vi "AlliGator NLSF & Phasor Multi-ROI Analysis Dialog.vi"(0 "Dialog Type":T22, 11 "error in (no error)":errorcluster) -> (1 "Dataset Loading & Pre-processing Options":T3={"Data Information"={"Gates to Skip"={"Start"=0, "End"=0}, "# Gates"=1, "Gate Step"=1, "Gate Duration"=3e-10, "Gate Separation"=4e-11, "Pile-up Correction"=FALSE, "Pixel Well Capacity"=1, "Define Gates to"=enum."Skip", "Gates to Keep"={"First"=0, "Last"=0}, "Laser Period"=0.0, "SYNC Period"=0.0, "Channel Name"=0, "Channel Arithmetic"=enum."None", "Background File Subtraction"=FALSE, "Background Scaling Factor"=1.0, "Background File"=path "", "Background Pile-up Correction"=FALSE, "Background Pixel Well Capacity"=1, "Dataset Scaling Factor"=1.0}, "Source Image Settings"={"Low Count Pixels Rejection Options"={"Background Low Threshold Factor"=0.0, "Fixed Low Background Threshold"=20000.0, "Reject Low Count Pixels"=FALSE, "Low Percentile"=0.0}, "High Count Pixels Rejection Options"={"Background High Threshold Factor"=0.0, "Fixed High Background Threshold"=1.0, "Reject High Count Pixels"=FALSE, "High Percentile"=100.0}, "Peak Threshold"=500.0, "Intensity Threshold"=500.0, "Image Smoothing Options"={"Use Image Smoothing"=FALSE, "Kernel Type"=enum."Bilinear", "Bin"=1, "Algorithm"=enum."Rapid"}, "Image Binning Options"={"Use Image Binning"=FALSE, "X Bin"=1, "Y Bin"=1}}, "Decay Preprocessing Options & Parameters"={"Background Subtraction Parameters"={"Background Definition Range"={"Min Gate"=0.0, "Max Gate"=0.0}, "Baseline Subtraction Method"=enum."Mean", "Background Subtraction?"=FALSE, "Background File"=path "", "Background Constant"=0.0, "Background Scaling Factor"=1.0, "Background Pile-up Correction"=FALSE, "Background Pixel Well Capacity"=1}, "Decay Preprocessing Parameters"={"Background Subtraction"=FALSE, "Straighten Decay"=FALSE, "Reverse Gates"=FALSE, "1-Normalized Decay"=FALSE, "Smoothen Decay"=FALSE, "Smoothing Parameter"=0.0, "Shift Decay"=FALSE, "Decay Shift Parameters"={"Type"=enum."Default", "Shift"=0.0, "Threshold"=0.0, "Rotate"=FALSE}, "Extrapolate Decay"=FALSE, "Additional Points"=0, "Head Fraction"=0.0, "Pixel-Normalize Decay"=FALSE, "Use Periodicity"=FALSE, "Use Cursors"=FALSE, "Tail Fraction"=0.0, "Use Decay Pre-Processing"=TRUE, "Fold Decay"=FALSE, "# Folds"=1, "[0-1]-Normalized Decay"=FALSE}, "Preprocessing Steps Order"=[]}, "Clear Phasor Graph"=FALSE} {"Decay Preprocessing Options & Parameters"."Decay Preprocessing Parameters"."# Folds" min=1; "Decay Preprocessing Options & Parameters"."Background Subtraction Parameters"."Background Pixel Well Capacity" min=1 step=1; "Source Image Settings"."Image Binning Options"."Y Bin" min=1; "Source Image Settings"."Image Binning Options"."X Bin" min=1; "Source Image Settings"."Image Smoothing Options"."Bin" min=1; "Source Image Settings"."High Count Pixels Rejection Options"."High Percentile" min=0.0 max=100.0; "Source Image Settings"."Low Count Pixels Rejection Options"."Low Percentile" min=0.0 max=100.0; "Data Information"."Background Pixel Well Capacity" min=1 step=1; "Data Information"."Channel Name" items=["Bottom INT Gate", "Bottom G2 Gate"]; "Data Information"."SYNC Period" min=0.0 format="%#.3g"; "Data Information"."Laser Period" min=0.0 format="%#.3g"; "Data Information"."Pixel Well Capacity" min=1 step=1; "Data Information"."# Gates" min=1 step=1; "Data Information"."Gate Step" min=1 step=1; "Data Information"."Gate Duration" min=0.0 format="%#.3g"; "Data Information"."Gate Separation" min=0.0 format="%#.3g"}, 2 "IRF Loading & Pre-processing Options":T3={"Data Information"={"Gates to Skip"={"Start"=0, "End"=0}, "# Gates"=1, "Gate Step"=1, "Gate Duration"=3e-10, "Gate Separation"=4e-11, "Pile-up Correction"=FALSE, "Pixel Well Capacity"=1, "Define Gates to"=enum."Skip", "Gates to Keep"={"First"=0, "Last"=0}, "Laser Period"=0.0, "SYNC Period"=0.0, "Channel Name"=0, "Channel Arithmetic"=enum."None", "Background File Subtraction"=FALSE, "Background Scaling Factor"=1.0, "Background File"=path "", "Background Pile-up Correction"=FALSE, "Background Pixel Well Capacity"=1, "Dataset Scaling Factor"=1.0}, "Source Image Settings"={"Low Count Pixels Rejection Options"={"Background Low Threshold Factor"=0.0, "Fixed Low Background Threshold"=20000.0, "Reject Low Count Pixels"=FALSE, "Low Percentile"=0.0}, "High Count Pixels Rejection Options"={"Background High Threshold Factor"=0.0, "Fixed High Background Threshold"=1.0, "Reject High Count Pixels"=FALSE, "High Percentile"=100.0}, "Peak Threshold"=500.0, "Intensity Threshold"=500.0, "Image Smoothing Options"={"Use Image Smoothing"=FALSE, "Kernel Type"=enum."Bilinear", "Bin"=1, "Algorithm"=enum."Rapid"}, "Image Binning Options"={"Use Image Binning"=FALSE, "X Bin"=1, "Y Bin"=1}}, "Decay Preprocessing Options & Parameters"={"Background Subtraction Parameters"={"Background Definition Range"={"Min Gate"=0.0, "Max Gate"=0.0}, "Baseline Subtraction Method"=enum."Mean", "Background Subtraction?"=FALSE, "Background File"=path "", "Background Constant"=0.0, "Background Scaling Factor"=1.0, "Background Pile-up Correction"=FALSE, "Background Pixel Well Capacity"=1}, "Decay Preprocessing Parameters"={"Background Subtraction"=FALSE, "Straighten Decay"=FALSE, "Reverse Gates"=FALSE, "1-Normalized Decay"=FALSE, "Smoothen Decay"=FALSE, "Smoothing Parameter"=0.0, "Shift Decay"=FALSE, "Decay Shift Parameters"={"Type"=enum."Default", "Shift"=0.0, "Threshold"=0.0, "Rotate"=FALSE}, "Extrapolate Decay"=FALSE, "Additional Points"=0, "Head Fraction"=0.0, "Pixel-Normalize Decay"=FALSE, "Use Periodicity"=FALSE, "Use Cursors"=FALSE, "Tail Fraction"=0.0, "Use Decay Pre-Processing"=TRUE, "Fold Decay"=FALSE, "# Folds"=1, "[0-1]-Normalized Decay"=FALSE}, "Preprocessing Steps Order"=[]}, "Clear Phasor Graph"=FALSE} {"Decay Preprocessing Options & Parameters"."Decay Preprocessing Parameters"."# Folds" min=1; "Decay Preprocessing Options & Parameters"."Background Subtraction Parameters"."Background Pixel Well Capacity" min=1 step=1; "Source Image Settings"."Image Binning Options"."Y Bin" min=1; "Source Image Settings"."Image Binning Options"."X Bin" min=1; "Source Image Settings"."Image Smoothing Options"."Bin" min=1; "Source Image Settings"."High Count Pixels Rejection Options"."High Percentile" min=0.0 max=100.0; "Source Image Settings"."Low Count Pixels Rejection Options"."Low Percentile" min=0.0 max=100.0; "Data Information"."Background Pixel Well Capacity" min=1 step=1; "Data Information"."Channel Name" items=["Bottom INT Gate", "Bottom G2 Gate"]; "Data Information"."SYNC Period" min=0.0 format="%#.3g"; "Data Information"."Laser Period" min=0.0 format="%#.3g"; "Data Information"."Pixel Well Capacity" min=1 step=1; "Data Information"."# Gates" min=1 step=1; "Data Information"."Gate Step" min=1 step=1; "Data Information"."Gate Duration" min=0.0 format="%#.3g"; "Data Information"."Gate Separation" min=0.0 format="%#.3g"}, 3 "OK":bool, 4 "IRF File":path, 6 "Dataset File":path, 8 "ROI File":path, 10 "Decay Fit Parameters to Save":T23[](array[typedef]), 12 "Phasor Parameters Scatter Plots":T1[](array[typedef]), 13 "Bins Array":dbl[](array[numeric]), 14 "Results Folder":path, 15 "error out":errorcluster)   [LabVIEW 2021, in "AlliGator Scripts.lvlib"]
doc: "Dialog window to set up a multi-ROIs single-pixel NLSF analysis of a FLI dataset."
uses:
  AlliGator Scripts.lvlib
  Fits/IRF(X)PSED/Decay Fit Parameters & Derived Quantities List.ctl
  AlliGator Data Load & Process Options.ctl
  AlliGator Data Information.ctl
  AlliGator Gates to Skip.ctl
  AlliGator Define Gates to.ctl
  AlliGator Gates to Keep.ctl
  AlliGator Gate Arithmetic.ctl
  AlliGator Source Image Settings.ctl
  AlliGator Low Count Pixels Rejection Options.ctl
  AlliGator High Count Pixels Rejection Options.ctl
  AlliGator Image Smoothing Options.ctl
  Arrays/Kernel Type.ctl
  Arrays/Smoothing Algorithm.ctl
  AlliGator Image Binning Options.ctl
  AlliGator Decay Preprocessing Options.ctl
  AlliGator Background Subtraction Parameters.ctl
  AlliGator Baseline Subtraction Method.ctl
  AlliGator Decay Preprocessing Parameters.ctl
  Graphs/XY Graph/XY Graph Plot Shift Parameters.ctl
  Graphs/XY Graph/XY Graph Plot Shift Method.ctl
  AlliGator Multi-ROIs Dialog Type.ctl
  AlliGator Phasor Plot Scatter Plot Parameters.ctl
  AlliGator Phasor Graph Parameter List.ctl
  84fa21cc-6b70-40ff-a749-33f909e19637.vi
  Error/Error.lvlib
  Fits/Fits.lvlib
  AlliGator Decay Analysis.lvlib
  AlliGator Settings.lvlib
  Arrays/Arrays.lvlib
  AlliGator Source Image.lvlib
  AlliGator Decay Preprocessing.lvlib
  Graphs/XY Graph/XY Graph Add-Ons.lvlib
  AlliGator Phasor Graph.lvlib
panel:
  in  "Clear Phasor Graph":bool
  in  "Save Results":bool
  in  "Phasor Parameters Scatter Plots":T1[](array[typedef])
  in  "Tab Control":enum32{"IRF Options", "Dataset Options"}(tab)
  out "Dataset Settings Saved":bool
  in  "Set Dataset Parameters":bool
  in  "Save Script":bool
  in  "Load Script":bool
  out "IRF Settings Saved":bool
  out "Message":string
  in  "Set IRF Parameters":bool
  in  "Bins":dbl[](array[numeric])
  in  "Results Folder:":path caption="Dataset File"
  in  "Decay Fit Parameters to save:":T23[](array[typedef])
  in  "ROI File:":path caption="Dataset File"
  in  "Dataset File:":path caption="Dataset File"
  in  "IRF File:":path caption="IRF File"
  in  "Cancel":bool
  in  "Run Script":bool
  in  "Use IRF Dataset":bool
  # "vs"
  # "vs"
  # "Gates Characteristics"
  # "Background File Subtraction"
  # "Gates Characteristics"
  # "Background File Subtraction"
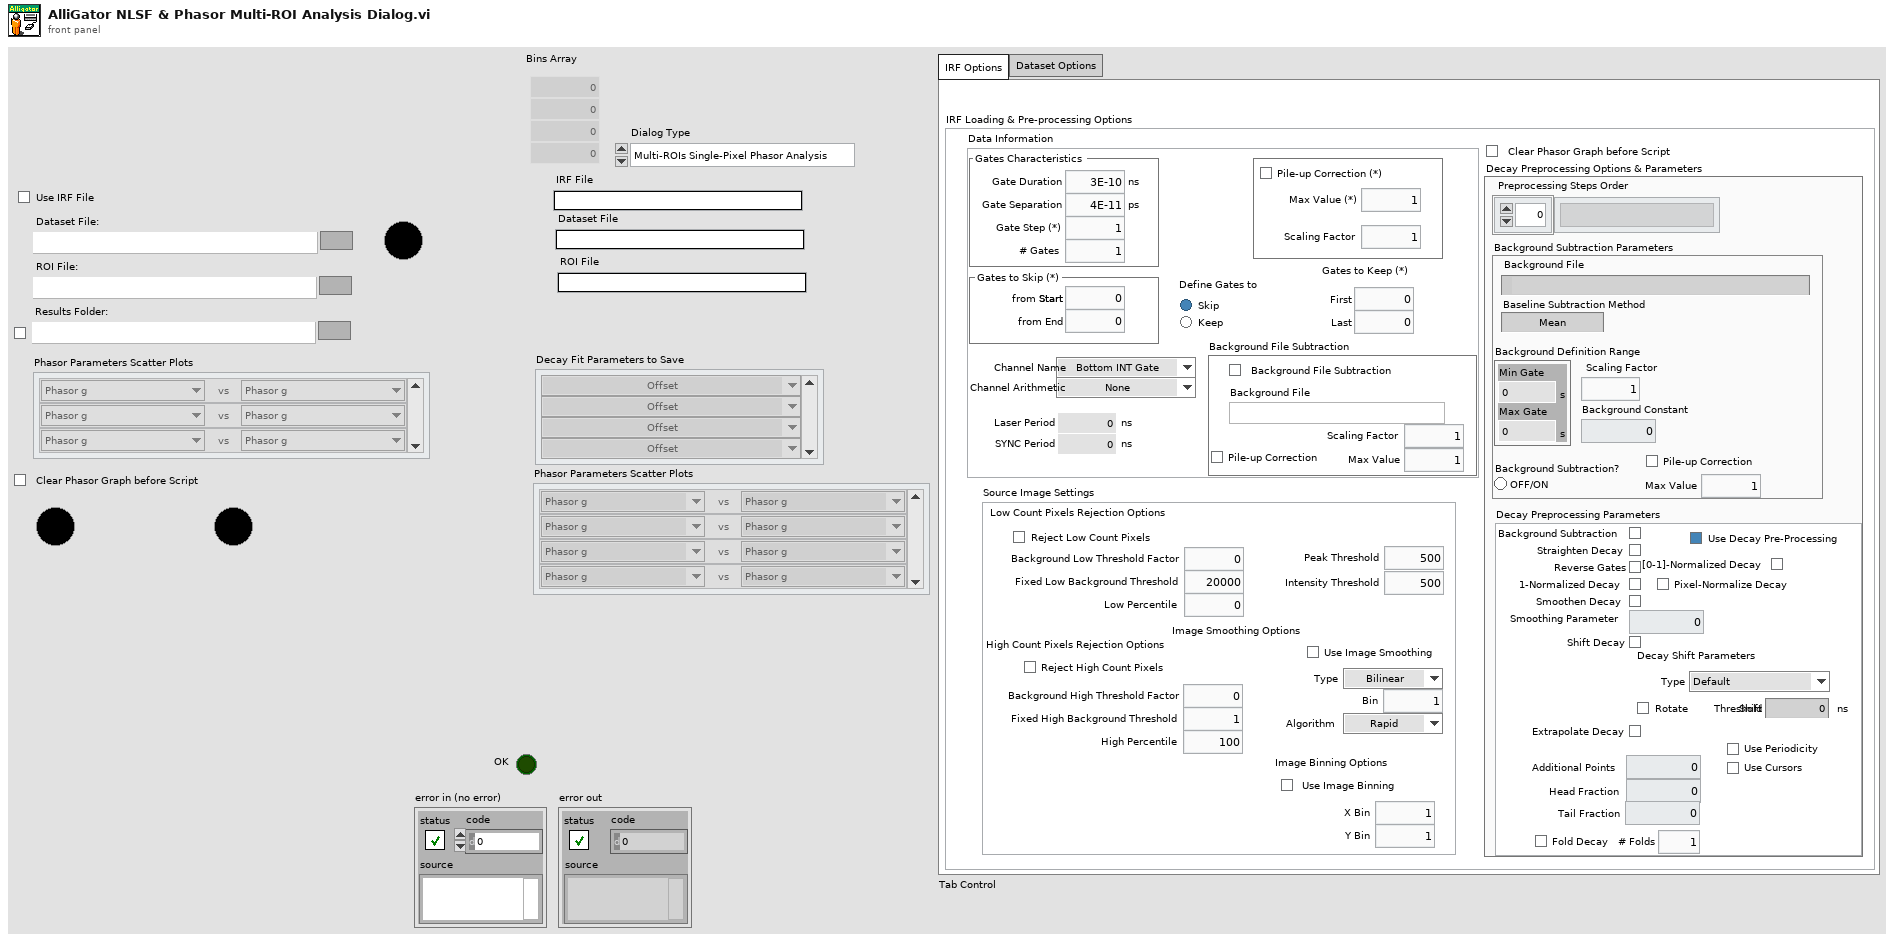
[diagram p1: front panel]
types:
  T1 = typedef "AlliGator Phasor Graph.lvlib/AlliGator Phasor Plot Scatter Plot Parameters.ctl" = cluster{"Parameter 2":T2, "Parameter 1":T2}
  T2 = typedef "AlliGator Phasor Graph.lvlib/AlliGator Phasor Graph Parameter List.ctl" = enum16{"Time Stamp", "Index", "Phasor Parameters", "Phasor g", "Phasor s", "Phasor phi", "Phasor m", "Modulus Lifetime", "Phase Lifetime", "ROI Parameters", "ROI Center x", "ROI Center y", "ROI # pixels ", "Decay Parameters", "Intensity", "Background/Gate", "Intensity - Background", "Fitted Lifetime", "Fitted Intensity", "Phasor Ratio Parameters", "Amplitude Phasor Ratio", "Intensity Phasor Ratio", "Amplitude-Averaged Lifetime", "Intensity-Averaged Lifetime", "-", "Phasor Parameters SDV", "Phasor g SDV", "Phasor s SDV", "Phasor phi SDV", "Phasor m SDV", "Phase Lifetime SDV", "Modulus Lifetime SDV", "Phasor Ratio Parameters SDV", "Amplitude Phasor Ratio SDV", "Intensity Phasor Ratio SDV", "Amplitude-Averaged Lifetime SDV", "Intensity-Averaged Lifetime SDV"}
  T3 = typedef "AlliGator Scripts.lvlib/AlliGator Data Load & Process Options.ctl" = cluster{"Data Information":T4, "Source Image Settings":T9, "Decay Preprocessing Options & Parameters":T16, "Clear Phasor Graph":bool}
  T4 = typedef "AlliGator Scripts.lvlib/AlliGator Data Information.ctl" = cluster{"Gates to Skip":T5, "# Gates":u32, "Gate Step":u32, "Gate Duration":dbl[unit], "Gate Separation":dbl[unit], "Pile-up Correction":bool, "Pixel Well Capacity":u32, "Define Gates to":T6, "Gates to Keep":T7, "Laser Period":dbl[unit], "SYNC Period":dbl[unit], "Channel Name":u16, "Channel Arithmetic":T8, "Background File Subtraction":bool, "Background Scaling Factor":dbl, "Background File":path, "Background Pile-up Correction":bool, "Background Pixel Well Capacity":u32, "Dataset Scaling Factor":dbl}
  T5 = typedef "AlliGator Decay Analysis.lvlib/AlliGator Gates to Skip.ctl" = cluster{"Start":u32, "End":u32}
  T6 = typedef "AlliGator Settings.lvlib/AlliGator Define Gates to.ctl" = enum32{"Skip", "Keep"}
  T7 = typedef "AlliGator Settings.lvlib/AlliGator Gates to Keep.ctl" = cluster{"First":u32, "Last":u32}
  T8 = typedef "AlliGator Settings.lvlib/AlliGator Gate Arithmetic.ctl" = enum16{"None", "INT-G2", "G2/INT*<INT>", "(1 - G2/INT)*<INT>"}
  T9 = typedef "AlliGator Scripts.lvlib/AlliGator Source Image Settings.ctl" = cluster{"Low Count Pixels Rejection Options":T10, "High Count Pixels Rejection Options":T11, "Peak Threshold":dbl, "Intensity Threshold":dbl, "Image Smoothing Options":T12, "Image Binning Options":T15}
  T10 = typedef "AlliGator Settings.lvlib/AlliGator Low Count Pixels Rejection Options.ctl" = cluster{"Background Low Threshold Factor":dbl, "Fixed Low Background Threshold":dbl, "Reject Low Count Pixels":bool, "Low Percentile":dbl}
  T11 = typedef "AlliGator Settings.lvlib/AlliGator High Count Pixels Rejection Options.ctl" = cluster{"Background High Threshold Factor":dbl, "Fixed High Background Threshold":dbl, "Reject High Count Pixels":bool, "High Percentile":dbl}
  T12 = typedef "AlliGator Settings.lvlib/AlliGator Image Smoothing Options.ctl" = cluster{"Use Image Smoothing":bool, "Kernel Type":T13, "Bin":i32, "Algorithm":T14}
  T13 = typedef "Arrays.lvlib/Kernel Type.ctl" = enum16{"Uniform", "Bilinear", "Gaussian"}
  T14 = typedef "Arrays.lvlib/Smoothing Algorithm.ctl" = enum16{"Rapid", "Thorough"}
  T15 = typedef "AlliGator Source Image.lvlib/AlliGator Image Binning Options.ctl" = cluster{"Use Image Binning":bool, "X Bin":i32, "Y Bin":i32}
  T16 = typedef "AlliGator Decay Analysis.lvlib/AlliGator Decay Preprocessing.lvlib/AlliGator Decay Preprocessing Options.ctl" = cluster{"Background Subtraction Parameters":T17, "Decay Preprocessing Parameters":T19, "Preprocessing Steps Order":string[]}
  T17 = typedef "AlliGator Decay Analysis.lvlib/AlliGator Decay Preprocessing.lvlib/AlliGator Background Subtraction Parameters.ctl" = cluster{"Background Definition Range":cluster{"Min Gate":dbl[unit], "Max Gate":dbl[unit]}, "Baseline Subtraction Method":T18, "Background Subtraction?":bool, "Background File":path, "Background Constant":dbl, "Background Scaling Factor":dbl, "Background Pile-up Correction":bool, "Background Pixel Well Capacity":u32}
  T18 = typedef "AlliGator Decay Analysis.lvlib/AlliGator Decay Preprocessing.lvlib/AlliGator Baseline Subtraction Method.ctl" = enum16{"Mean", "Min", "Square Gated Single-Exponential", "File", "Constant"}
  T19 = typedef "AlliGator Decay Analysis.lvlib/AlliGator Decay Preprocessing.lvlib/AlliGator Decay Preprocessing Parameters.ctl" = cluster{"Background Subtraction":bool, "Straighten Decay":bool, "Reverse Gates":bool, "1-Normalized Decay":bool, "Smoothen Decay":bool, "Smoothing Parameter":dbl, "Shift Decay":bool, "Decay Shift Parameters":T20, "Extrapolate Decay":bool, "Additional Points":u32, "Head Fraction":dbl, "Pixel-Normalize Decay":bool, "Use Periodicity":bool, "Use Cursors":bool, "Tail Fraction":dbl, "Use Decay Pre-Processing":bool, "Fold Decay":bool, "# Folds":u32, "[0-1]-Normalized Decay":bool}
  T20 = typedef "XY Graph Add-Ons.lvlib/XY Graph Plot Shift Parameters.ctl" = cluster{"Type":T21, "Shift":dbl[unit], "Threshold":dbl, "Rotate":bool}
  T21 = typedef "XY Graph Add-Ons.lvlib/XY Graph Plot Shift Method.ctl" = enum16{"Default", "CFD", "Threshold", "Cross-Correlation"}
  T22 = typedef "AlliGator Scripts.lvlib/AlliGator Multi-ROIs Dialog Type.ctl" = enum16{"Multi-ROIs Single-Pixel Phasor Analysis", "Multi-ROIs Single-Pixel NLSF Analysis", "Export ROI Fit Parameters as ASCII"}
  T23 = typedef "Fits.lvlib/Decay Fit Parameters & Derived Quantities List.ctl" = enum16{"Offset", "Baseline", "A_1", "tau_1", "A_2", "tau_2", "<tau>_a", "f1_a", "f2_a", "<tau>_i", "f1_i", "f2_i", "-", "R^2", "Chi^2"}
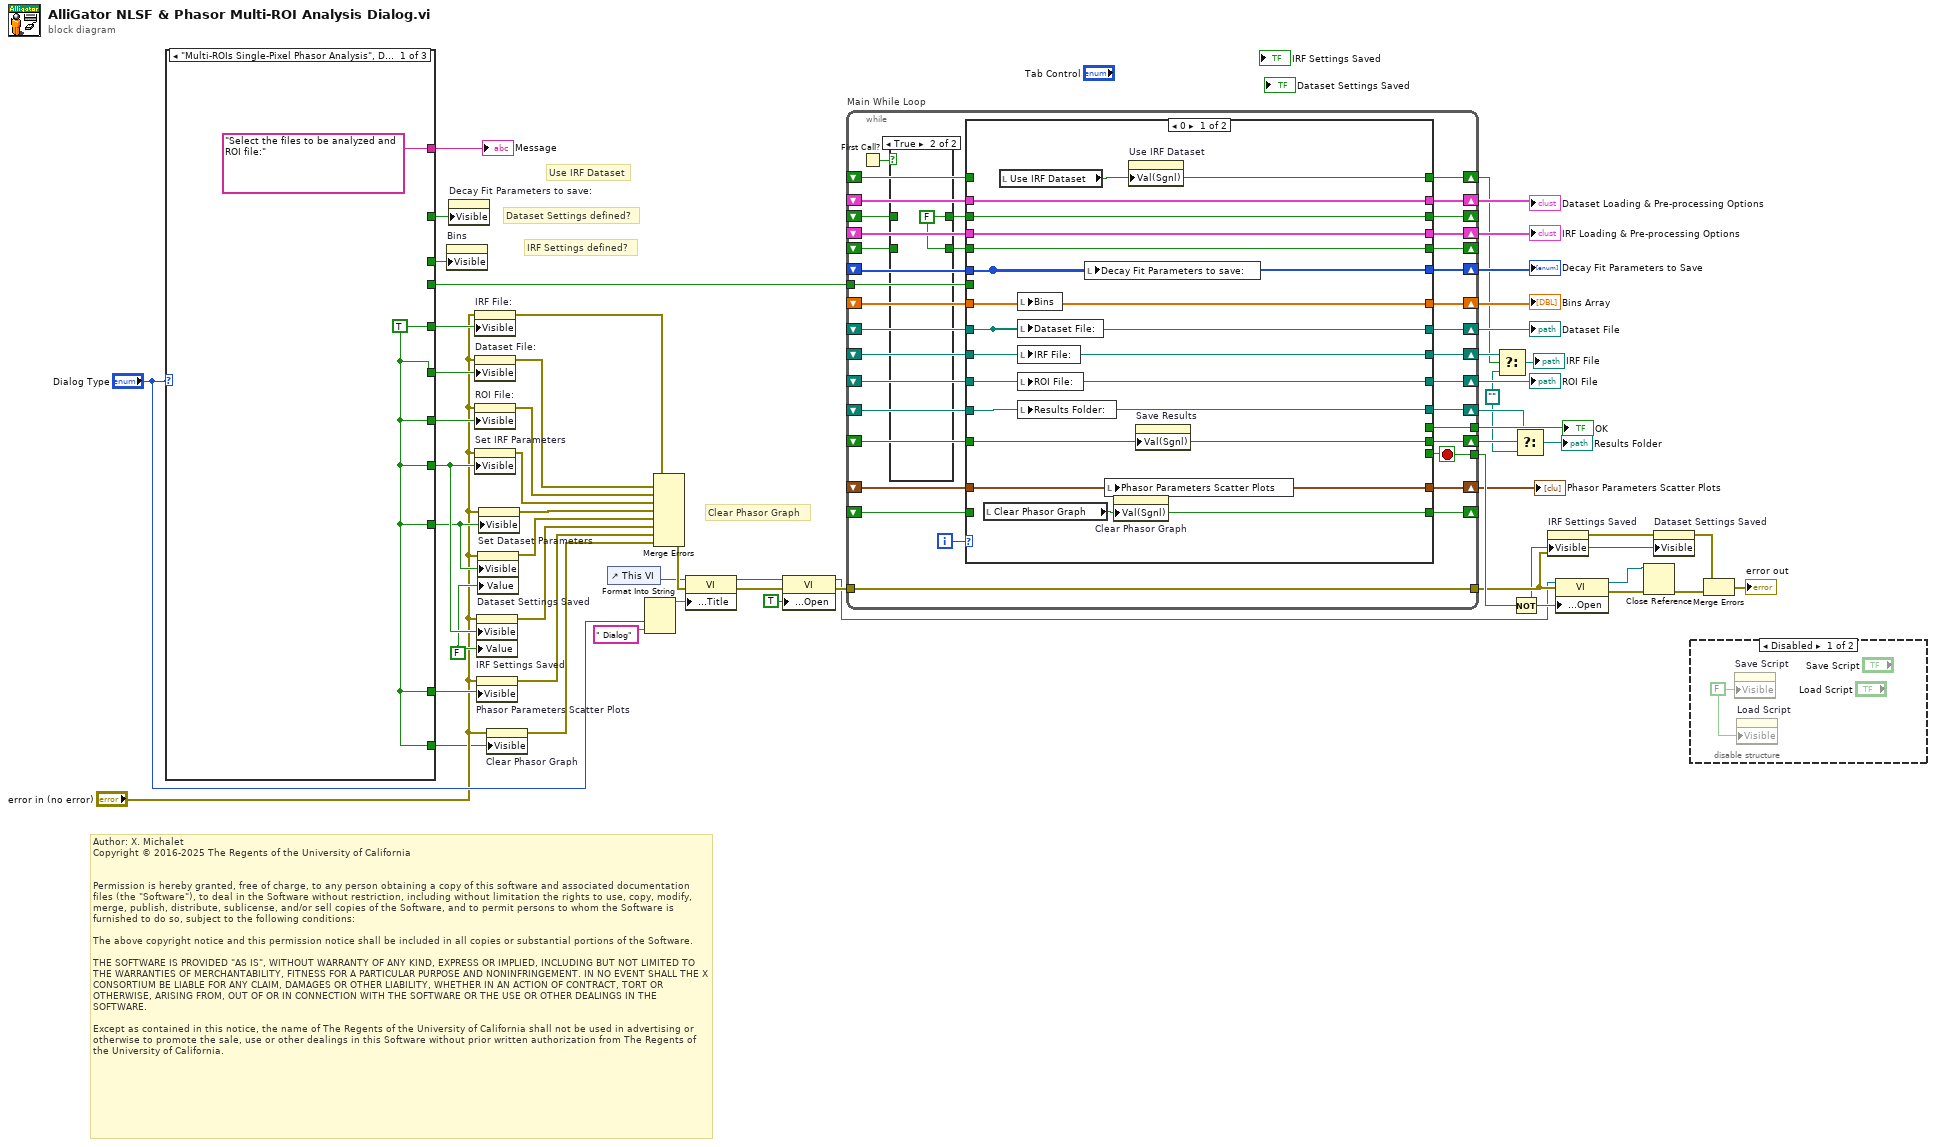
[diagram p0: block diagram]
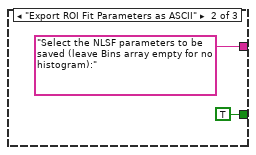
[diagram p3: hidden frame]
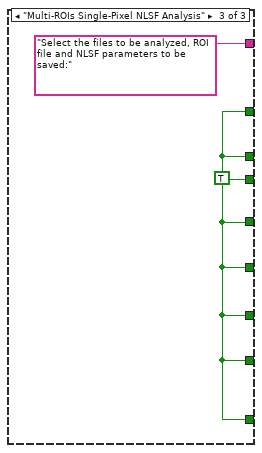
[diagram p4: hidden frame]
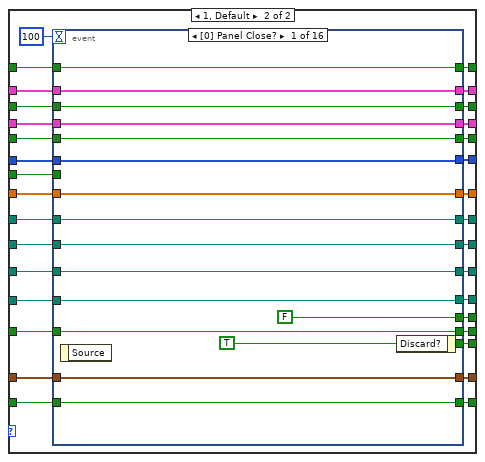
[diagram p6: hidden frame]
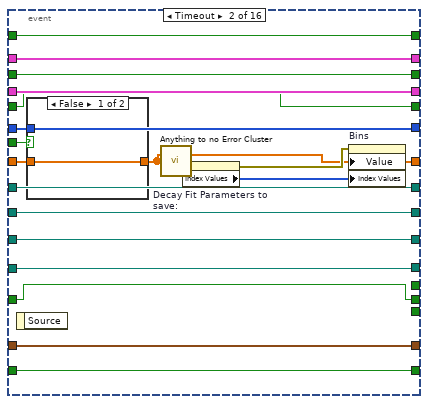
[diagram p7: hidden frame]
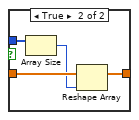
[diagram p8: hidden frame]
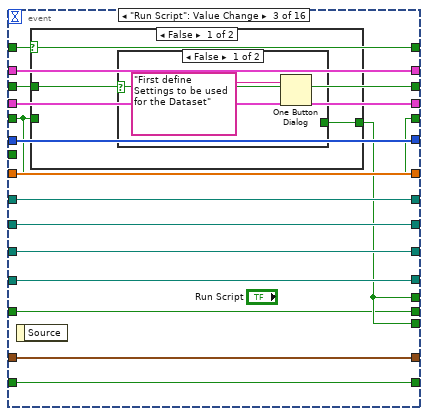
[diagram p9: hidden frame]
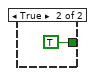
[diagram p10: hidden frame]
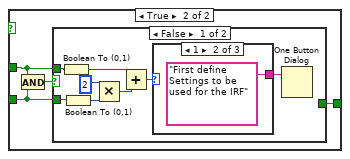
[diagram p11: hidden frame]
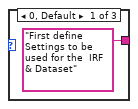
[diagram p12: hidden frame]
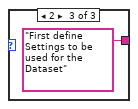
[diagram p13: hidden frame]
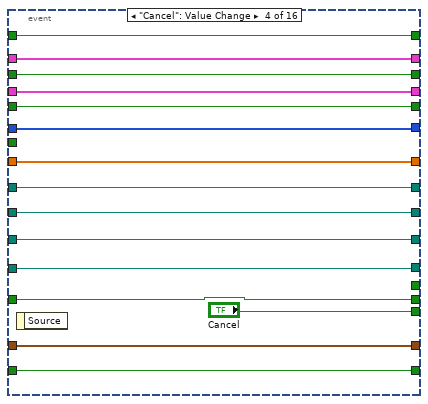
[diagram p15: hidden frame]
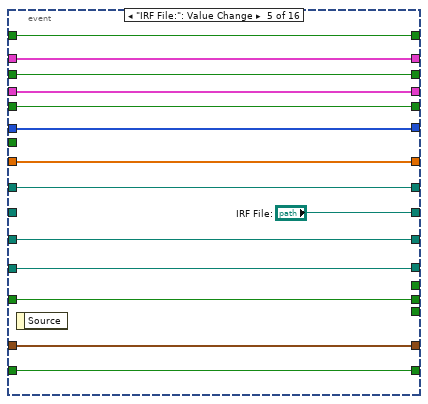
[diagram p16: hidden frame]
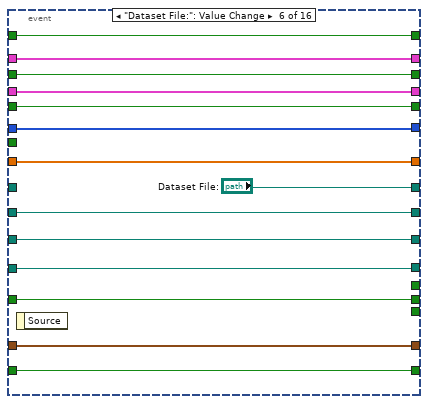
[diagram p17: hidden frame]
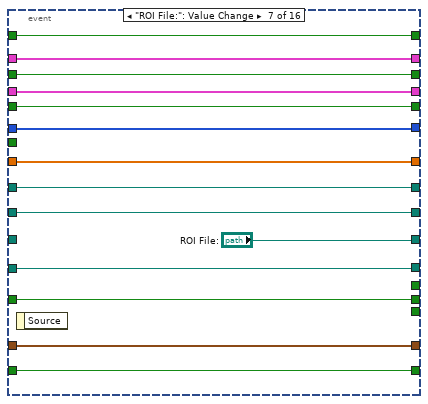
[diagram p18: hidden frame]
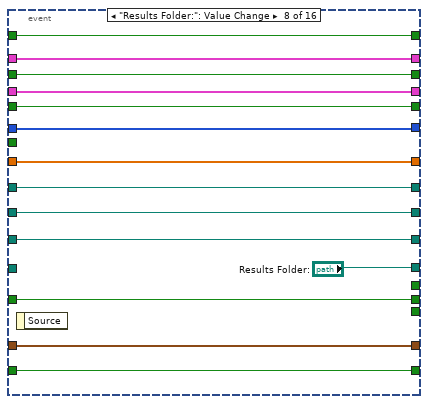
[diagram p19: hidden frame]
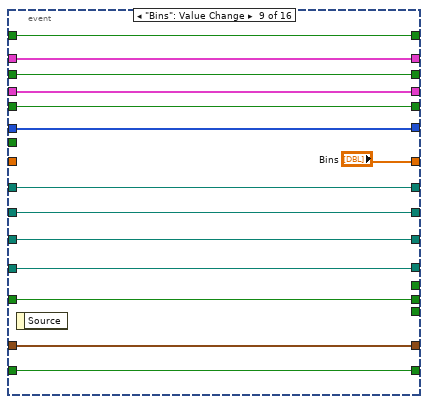
[diagram p20: hidden frame]
diagram:
  w15 = path ""
  w23 = FALSE ("Dataset Options Saved")
  # "Author: X. Michalet\nCopyright © 2016-2025 The Regents of the University of California\n \n\nPermission is hereby granted, free of charge, to any person obtaining a copy of this software and associated documentation files (the \"Software\"), to deal in the Software without restriction, including without limitation the rights to use, copy, modify, merge, publish, distribute, sublicense, and/or sell copies of the Software, and to permit persons to whom the Software is furnished to do so, subject to the following conditions:\n\nThe above copyright notice and this permission notice shall be included in all copies or substantial portions of the Software.\n\nTHE SOFTWARE IS PROVIDED \"AS IS\", WITHOUT WARRANTY OF ANY KIND, EXPRESS OR IMPLIED, INCLUDING BUT NOT LIMITED TO THE WARRANTIES OF MERCHANTABILITY, FITNESS FOR A PARTICULAR PURPOSE AND NONINFRINGEMENT. IN NO EVENT SHALL THE X CONSORTIUM BE LIABLE FOR ANY CLAIM, DAMAGES OR OTHER LIABILITY, WHETHER IN AN ACTION OF CONTRACT, TORT OR OTHERWISE, ARISING FROM, OUT OF OR IN CONNECTION WITH THE SOFTWARE OR THE USE OR OTHER DEALINGS IN THE SOFTWARE.\n\nExcept as contained in this notice, the name of The Regents of the University of California shall not be used in advertising or otherwise to promote the sale, use or other dealings in this Software without prior written authorization from The Regents of the University of California."
  # "Clear Phasor Graph"
  # "Use IRF Dataset"
  # "IRF Settings defined?"
  # "Dataset Settings defined?"
  n1 = case shown="\"Multi-ROIs Single-Pixel Phasor Analysis\", Default" "Dialog Type" {
    tunnel: ["Select the files to be analyzed and ROI file:" ("Message") "Select the NLSF parameters to be  saved (leave Bins array empty for no histogram):" ("Message") "Select the files to be analyzed, ROI file and NLSF parameters to be saved:" ("Message")] -> w46
    tunnel: [_ _ w61] -> w45
    tunnel: [w57 _ w61] -> w44
    tunnel: [w57 _ w61] -> w43
    tunnel: [w57 _ w61] -> w42
    tunnel: [w57 _ w61] -> w25
    tunnel: [_ TRUE ("Front Panel Window:Open") w61] -> w36
    tunnel: [_ _ w61] -> w35
    tunnel: [w57 _ w61] -> w24
    tunnel: [w57 _ _] -> w18
    tunnel: [w57 _ _] -> w1
    frame "Multi-ROIs Single-Pixel Phasor Analysis", Default {
      w57 = TRUE ("Visible")
    }
    frame "Export ROI Fit Parameters as ASCII" {
    }
    frame "Multi-ROIs Single-Pixel NLSF Analysis" {
      w61 = TRUE ("Front Panel Window:Open")
    }
  }
  "Message" <- w46
  n2 = property on="Bins" class="Arr (strict)"("Visible"=w35) -> ()  [unwired: 2 in, 2 out]
  n3 = property on="Decay Fit Parameters to save:" class="Arr (strict)"("Visible"=w36) -> ()  [unwired: 2 in, 2 out]
  n4 = property on="IRF File:" class="Path"(error in="error in (no error)", "Visible"=w44) -> (error out=w41:errorcluster)  [unwired: 1 in, 1 out]
  n5 = property on="Dataset File:" class="Path"(error in="error in (no error)", "Visible"=w43) -> (error out=w39:errorcluster)  [unwired: 1 in, 1 out]
  n6 = property on="ROI File:" class="Path"(error in="error in (no error)", "Visible"=w42) -> (error out=w38:errorcluster)  [unwired: 1 in, 1 out]
  n7 = property on="Set IRF Parameters" class="Bool"(error in="error in (no error)", "Visible"=w25) -> (error out=w37:errorcluster)  [unwired: 1 in, 1 out]
  n8 = property on="IRF Settings Saved" class="Bool (strict)"(error in="error in (no error)", "Visible"=w25, "Value"=w23) -> (error out=w26:errorcluster)  [unwired: 1 in, 1 out]
  n9 = property on="Phasor Parameters Scatter Plots" class="Arr (strict)"(error in="error in (no error)", "Visible"=w18) -> (error out=w3:errorcluster)  [unwired: 1 in, 1 out]
  n10 = property on="Dataset Settings Saved" class="Bool (strict)"(error in="error in (no error)", "Visible"=w24, "Value"=w23) -> (error out=w27:errorcluster)  [unwired: 1 in, 1 out]
  n11 = property on="Set Dataset Parameters" class="Bool"(error in="error in (no error)", "Visible"=w24) -> (error out=w31:errorcluster)  [unwired: 1 in, 1 out]
  n12 = property on="Clear Phasor Graph" class="Bool (strict)"(error in="error in (no error)", "Visible"=w1) -> (error out=w2:errorcluster)  [unwired: 1 in, 1 out]
  n13 = control-ref of="This VI"() -> (w12:refnum<vi>)
  n14 = Format Into String("Dialog Type", " Dialog" ("Front Panel Window:Title")) -> (resulting string=w10:string)  [unwired: 3 in, 1 out]
  n15 = Merge Errors(w41, w39, w38, w37, w31, w27, w26, w3, w2) -> (w40:errorcluster)
  n16 = property class="VI"(reference=w12, error in=w40, "Front Panel.Title"=w10) -> (reference out=w11:refnum<vi>, error out=w13:errorcluster)
  n17 = property class="VI"(reference=w11, error in=w13, "Front Panel Window:Open"=TRUE) -> (reference out=w7:refnum<vi>, error out=w56:errorcluster)
  n18 = while "Main While Loop" {
    tunnel: w56 -> [w98]
    tunnel: [w98] -> w34
    tunnel: [w97] -> w54
    tunnel: [w96] -> w53
    shift-right: [w95] -> w52
    shift-left: _ -> [w93]
    shift-right: [w94] -> w22
    shift-left: _ -> [w91]
    shift-right: [w92] -> w51
    shift-left: _ -> [w90]
    shift-right: [w88] -> w50
    shift-left: _ -> [w87]
    shift-right: [w85] -> w16
    shift-left: _ -> [w86]
    shift-right: [w84] -> w49
    shift-left: _ -> [w83]
    shift-right: [w82] -> w48
    shift-left: _ -> [w81]
    tunnel: w45 -> [w80]
    shift-right: [w79] -> w32
    shift-left: _ -> [w78]
    shift-right: [w77] -> w19
    shift-left: _ -> [w76]
    shift-right: [w75] -> w20
    shift-left: _ -> [w74]
    shift-right: [w67] -> _
    shift-left: _ -> [w72]
    shift-right: [w68] -> _
    shift-left: _ -> [w71]
    shift-right: [w65] -> w17
    shift-left: _ -> [w66]
    shift-right: [w63] -> _
    shift-left: _ -> [w64]
    i -> [w89]
    stop <- w96 stop-if-true
    n19 = First Call?() -> (First Call?: T/F=w73:bool)
    n20 = case shown="True" w73 {
      tunnel: w72 -> [w100 _]
      tunnel: [w100 w101] -> w70
      tunnel: [w99 w101] -> w69
      tunnel: w71 -> [w99 _]
      frame False {
      }
      frame True {
        w101 = FALSE
      }
    }
    n21 = case shown="0" w89 {
      tunnel: [_ w147] -> w97
      tunnel: [_ w146] -> w96
      tunnel: [w115 w145] -> w95
      tunnel: [w113 w144] -> w94
      tunnel: w93 -> [w115 w143]
      tunnel: [w114 w142] -> w92
      tunnel: w91 -> [w113 w141]
      tunnel: w90 -> [w114 w140]
      tunnel: [w112 w139] -> w88
      tunnel: w87 -> [w112 w138]
      tunnel: w86 -> [w111 w136]
      tunnel: [w111 w137] -> w85
      tunnel: [w110 w135] -> w84
      tunnel: w83 -> [w110 w134]
      tunnel: [w107 w132] -> w82
      tunnel: w81 -> [w107 w131]
      tunnel: w80 -> [_ w130]
      tunnel: [w108 w129] -> w79
      tunnel: w78 -> [w108 w128]
      tunnel: [w109 w127] -> w77
      tunnel: w76 -> [w109 w126]
      tunnel: [w102 w125] -> w75
      tunnel: w74 -> [_ w124]
      tunnel: w70 -> [w106 w123]
      tunnel: w69 -> [w105 w122]
      tunnel: [w105 w121] -> w68
      tunnel: [w106 w120] -> w67
      tunnel: w66 -> [w104 w118]
      tunnel: [w104 w119] -> w65
      tunnel: w64 -> [_ w116]
      tunnel: [w103 w117] -> w63
      frame 0 {
        n22 = local read "Clear Phasor Graph"() -> (w103:bool)
        n23 = local read "Use IRF Dataset"() -> (w102:bool)
        n24 = local write "Bins"(w110) -> ()
        n25 = local write "Dataset File:"(w115) -> ()
        n26 = local write "IRF File:"(w113) -> ()
        n27 = local write "ROI File:"(w114) -> ()
        n28 = local write "Results Folder:"(w111) -> ()
        n29 = local write "Decay Fit Parameters to save:"(w112) -> ()
        n30 = local write "Phasor Parameters Scatter Plots"(w109) -> ()
        n31 = property on="Clear Phasor Graph" class="Bool (strict)"("Val(Sgnl)"=w103) -> ()  [unwired: 2 in, 2 out]
        n32 = property on="Use IRF Dataset" class="Bool (strict)"("Val(Sgnl)"=w102) -> ()  [unwired: 2 in, 2 out]
        n33 = property on="Save Results" class="Bool (strict)"("Val(Sgnl)"=w104) -> ()  [unwired: 2 in, 2 out]
      }
      frame 1, Default {
        n34 = event shown="[0] Panel Close?" {
          selector: _ -> [_ _ _ _ _ _ _ _ _ _ _ _ _ _ _ _]
          dyn-events: _ -> [_ _ _ _ _ _ _ _ _ _ _ _ _ _ _ _]
          timeout: 100 -> [_ _ _ _ _ _ _ _ _ _ _ _ _ _ _ _]
          tunnel: [w163 _ w191 "Cancel" _ _ _ _ _ _ _ _ _ _ _ _] -> w146
          tunnel: [FALSE ("OK") _ w191 _ _ _ _ _ _ _ _ _ _ _ _ _] -> w147
          tunnel: [w161 w182 w202 w236 w250 "Dataset File:" w279 w293 w307 w322 w338 w354 w368 w384 w399 w414] -> w145
          tunnel: [w160 w181 w201 w235 "IRF File:" w265 w278 w292 w306 w321 w337 w353 w367 w383 w398 w413] -> w144
          tunnel: w143 -> [w161 w182 w202 w236 w250 _ w279 w293 w307 w322 w338 w354 w368 w384 w399 w414]
          tunnel: [w159 w180 w200 w234 w249 w264 "ROI File:" w291 w305 w320 w336 w352 w366 w382 w397 w412] -> w142
          tunnel: w141 -> [w160 w181 w201 w235 _ w265 w278 w292 w306 w321 w337 w353 w367 w383 w398 w413]
          tunnel: w140 -> [w159 w180 w200 w234 w249 w264 _ w291 w305 w320 w336 w352 w366 w382 w397 w412]
          tunnel: [w158 w178 w199 w233 w248 w263 w277 w290 w304 w318 w335 w351 w365 w381 w396 w411] -> w139
          tunnel: w138 -> [w158 w178 w199 w233 w248 w263 w277 w290 w304 _ w335 w351 w365 w381 w396 w411]
          tunnel: [w157 w179 w198 w232 w247 w261 w275 "Results Folder:" w303 w317 w334 w350 w364 w380 w395 w410] -> w137
          tunnel: w136 -> [w157 w179 w198 w232 w247 w261 w275 _ w303 w317 w334 w350 w364 w380 w395 w410]
          tunnel: [w156 w173 w197 w231 w246 w260 w274 w288 "Bins" w316 w333 w349 w363 w379 w394 w409] -> w135
          tunnel: w134 -> [w156 w177 w197 w231 w246 w260 w274 w288 _ w316 w333 w349 w363 w379 w394 w409]
          tunnel: [w155 w172 w196 w230 w245 w259 w273 w287 w301 w315 w332 w345 w362 w378 w393 w408] -> w132
          tunnel: w131 -> [w155 w172 w196 w230 w245 w259 w273 w287 w301 w315 _ w345 w362 w378 w393 w408]
          tunnel: w130 -> [_ w171 _ _ _ _ _ _ _ _ _ _ _ _ _ _]
          tunnel: [w154 w170 w195 w229 w244 w258 w272 w286 w300 w314 w329 w346 w361 w377 w392 w401] -> w129
          tunnel: w128 -> [w154 w170 w195 w229 w244 w258 w272 w286 w300 w314 w329 _ w361 w377 w392 w402]
          tunnel: [w153 w169 w194 w228 w243 w257 w271 w285 w299 w313 w328 w344 "Phasor Parameters Scatter Plots" w376 w391 w407] -> w127
          tunnel: w126 -> [w153 w169 w194 w228 w243 w257 w271 w285 w299 w313 w328 w344 _ w376 w391 w407]
          tunnel: [w152 w168 w193 w227 w242 w256 w270 w284 w298 w312 w327 w343 w360 "Use IRF Dataset" w386 w406] -> w125
          tunnel: w124 -> [w152 w168 w193 w227 w242 w256 w270 w284 w298 w312 w327 w343 w360 _ w386 w406]
          tunnel: w123 -> [w150 w166 w192 w225 w240 w254 w268 w282 w296 w310 w325 _ w358 w371 w388 w404]
          tunnel: w122 -> [w151 w167 w190 w226 w241 w255 w269 w283 w297 w311 _ w342 w359 w372 w389 w405]
          tunnel: [w151 w167 w190 w226 w241 w255 w269 w283 w297 w311 TRUE ("Get (F)/Set") w342 w359 w372 w389 w405] -> w121
          tunnel: [w150 w166 w192 w225 w240 w254 w268 w282 w296 w310 w325 TRUE ("Get (F)/Set") w358 w371 w388 w404] -> w120
          tunnel: [w149 w165 w189 w224 w239 w253 w267 w281 w295 w309 w324 w340 w356 w370 "Save Results" w403] -> w119
          tunnel: w118 -> [w149 w165 w189 w224 w239 w253 w267 w281 w295 w309 w324 w340 w356 w370 _ w403]
          tunnel: [w148 w164 w188 w223 w238 w252 w266 w280 w294 w308 w323 w339 w355 w369 w385 "Clear Phasor Graph"] -> w117
          tunnel: w116 -> [w148 w164 w188 w223 w238 w252 w266 w280 w294 w308 w323 w339 w355 w369 w385 _]
          event Panel Close? {
            w163 = TRUE ("Discard?")
            n35 = event-data() -> ()  [unwired: 1 in, 1 out]
            n36 = event-data("Discard?"=w163) -> ()  [unwired: 1 in, 1 out]
          }
          event Timeout {
            n37 = event-data() -> ()  [unwired: 1 in, 1 out]
            n38 = case shown="False" w171 {
              tunnel: w178 -> [_ w187]
              tunnel: w177 -> [w183 w186]
              tunnel: [w183 w184] -> w173
              frame False {
              }
              frame True {
                n39 = Array Size(array=w187) -> (size(s)=w185:i32)
                n40 = Reshape Array(w186, w185) -> (w184:dbl[])
              }
            }
            n41 = call "Anything to no Error Cluster.vi"("Variant"=w173) -> ("Error Out"=w174:errorcluster)  [unwired: 8 in]
            n42 = property on="Decay Fit Parameters to save:" class="Arr (strict)"(error in=w174) -> (error out=w175:errorcluster, "Index Values"=w176:u32[])  [unwired: 1 in, 1 out]
            n43 = property on="Bins" class="Arr (strict)"(error in=w175, "Value"=w173, "Index Values"=w176) -> ()  [unwired: 1 in, 2 out]
          }
          event "Run Script": Value Change {
            n44 = event-data() -> ()  [unwired: 1 in, 1 out]
            n45 = case shown="False" w193 {
              tunnel: w192 -> [w204 w208]
              tunnel: [w203 w209] -> w191
              tunnel: w190 -> [_ w207]
              frame False {
                n46 = case shown="False" w204 {
                  tunnel: [_ TRUE] -> w203
                  frame False {
                    n47 = One Button Dialog(message="First define Settings to be used for the Dataset") -> ()  [unwired: 1 in, 1 out]
                  }
                  frame True {
                  }
                }
              }
              frame True {
                n48 = And(x=w208, y=w207) -> (x .and. y?=w210:bool)
                n49 = case shown="False" w210 {
                  selector: w210 -> [_ w222]
                  tunnel: [_ w222] -> w209
                  tunnel: w208 -> [w218 _]
                  tunnel: w207 -> [w217 _]
                  frame False {
                    n50 = Boolean To (0,1)(Boolean=w218) -> (0, 1=w214:i16)
                    n51 = Boolean To (0,1)(Boolean=w217) -> (0, 1=w216:i16)
                    n52 = Multiply(x=i16 2, y=w216) -> (x*y=w213:i16)
                    n53 = Add(x=w214, y=w213) -> (x+y=w212:i16)
                    n54 = case shown="1" w212 {
                      tunnel: ["First define Settings to be used for the  IRF & Dataset" ("message") "First define Settings to be used for the IRF" ("message") "First define Settings to be used for the Dataset" ("message")] -> w211
                      frame 0, Default {
                      }
                      frame 1 {
                      }
                      frame 2 {
                      }
                    }
                    n55 = One Button Dialog(message=w211) -> ()  [unwired: 1 in, 1 out]
                  }
                  frame True {
                  }
                }
              }
            }
          }
          event "Cancel": Value Change {
            n56 = event-data() -> ()  [unwired: 1 in, 1 out]
          }
          event "IRF File:": Value Change {
            n57 = event-data() -> ()  [unwired: 1 in, 1 out]
          }
          event "Dataset File:": Value Change {
            n58 = event-data() -> ()  [unwired: 1 in, 1 out]
          }
          event "ROI File:": Value Change {
            n59 = event-data() -> ()  [unwired: 1 in, 1 out]
          }
          event "Results Folder:": Value Change {
            n60 = event-data() -> ()  [unwired: 1 in, 1 out]
          }
          event "Bins": Value Change {
            n61 = event-data() -> ()  [unwired: 1 in, 1 out]
          }
          event "Decay Fit Parameters to save:": Value Change {
            n62 = event-data() -> ()  [unwired: 1 in, 1 out]
            n63 = call "Remove Duplicates From 1D Array.vim"("array"="Decay Fit Parameters to save:") -> ("array with duplicates removed"=w318:T23[])  [unwired: 10 in]
            n64 = property on="Decay Fit Parameters to save:" class="Arr (strict)"("Value"=w318) -> ()  [unwired: 2 in, 2 out]
          }
          event "Set IRF Parameters": Value Change {
            n65 = event-data() -> ()  [unwired: 1 in, 1 out]
            n66 = property on="IRF Settings Saved" class="Bool (strict)"("Value"="Set IRF Parameters", "Visible"="Set IRF Parameters") -> ()  [unwired: 2 in, 2 out]
            n67 = call "AlliGator Get-Set Loading & Pre-Processing Options.vi"("Get (F)/Set"=FALSE) -> ("Dataset Loading & Pre-processing Options (out)"=w332:T3)  [unwired: 9 in, 1 out]
          }
          event "Set Dataset Parameters": Value Change {
            n68 = event-data() -> ()  [unwired: 1 in, 1 out]
            n69 = property on="Dataset Settings Saved" class="Bool (strict)"("Value"="Set Dataset Parameters", "Visible"="Set Dataset Parameters") -> ()  [unwired: 2 in, 2 out]
            n70 = call "AlliGator Get-Set Loading & Pre-Processing Options.vi"("Get (F)/Set"=FALSE) -> ("Dataset Loading & Pre-processing Options (out)"=w346:T3)  [unwired: 9 in, 1 out]
          }
          event "Phasor Parameters Scatter Plots": Value Change {
            n71 = event-data() -> ()  [unwired: 1 in, 1 out]
          }
          event "Use IRF Dataset": Value Change {
            n72 = event-data() -> ("NewVal"=w375:bool)  [unwired: 1 in]
            n73 = property on="IRF File:" class="Path"("Visible"=w375) -> ()  [unwired: 2 in, 2 out]
            n74 = property on="Set IRF Parameters" class="Bool"("Visible"=w375) -> ()  [unwired: 2 in, 2 out]
            n75 = property on="IRF Settings Saved" class="Bool (strict)"("Visible"="Use IRF Dataset", "Value"=FALSE ("Visible")) -> ()  [unwired: 2 in, 2 out]
          }
          event "Save Results": Value Change {
            n76 = event-data() -> ("NewVal"=w390:bool)  [unwired: 1 in]
            n77 = property on="Results Folder" class="Path"("Visible"=w390) -> ()  [unwired: 2 in, 2 out]
          }
          event "Clear Phasor Graph": Value Change {
            n78 = event-data() -> ()  [unwired: 1 in, 1 out]
            n79 = Bundle By Name(cluster=w402, "Clear Phasor Graph"="Clear Phasor Graph") -> (w401:T3)
          }
        }
      }
    }
  }
  "OK" <- w54
  "Dataset File" <- w52
  "ROI File" <- w51
  "Decay Fit Parameters to Save" <- w50
  "Bins Array" <- w49
  "IRF Loading & Pre-processing Options" <- w48
  "Dataset Loading & Pre-processing Options" <- w32
  "Phasor Parameters Scatter Plots" <- w19
  n80 = Select(t=w22, s=w20, f=w15) -> (s? t:f=→"IRF File":path)
  n81 = Not(x=w53) -> (.not. x?=w29:bool)
  n82 = Select(t=w16, s=w17, f=w15) -> (s? t:f=→"Results Folder":path)
  n83 = property on="IRF Settings Saved" class="Bool (strict)"(error in=w34, "Visible"=w29) -> (error out=w30:errorcluster)  [unwired: 1 in, 1 out]
  n84 = property class="VI"(reference=w7, error in=w34, "Front Panel Window:Open"=w29) -> (reference out=w5:refnum<vi>, error out=w55:errorcluster)
  n85 = Close Reference(reference=w5, error in (no error)=w55) -> (error out=w6:errorcluster)
  n86 = property on="Dataset Settings Saved" class="Bool (strict)"(error in=w30, "Visible"=w29) -> (error out=w28:errorcluster)  [unwired: 1 in, 1 out]
  n87 = disable-structure shown="Disabled" {
    frame Disabled {
      w415 = FALSE ("Visible")
      n88 = property on="Save Script" class="Bool"("Visible"=w415) -> ()  [unwired: 2 in, 2 out]
      n89 = property on="Load Script" class="Bool"("Visible"=w415) -> ()  [unwired: 2 in, 2 out]
    }
    frame Enabled {
    }
  }
  n90 = Merge Errors(w28, w6) -> (→"error out":errorcluster)
